vi "Test Create Report.vi"(8 "error in (no error)":errorcluster, 11 "XML Report Test in":refnum<class "Text Report Test.lvclass">) -> (0 "error out":errorcluster, 3 "XML Report Test out":refnum<class "Text Report Test.lvclass">)   [LabVIEW 2020, in "Text Report Test.lvclass"]
uses:
  Text Report Test.lvclass
  C:/Program Files (x86)/National Instruments/LabVIEW 2020/vi.lib/Astemes/LUnit/Test Case.lvclass
  Text Report Test.lvclass/Text Report Test.ctl
  <vilib>/Astemes/LUnit/Test Case.lvclass/Test Case.ctl
  <vilib>/Astemes/LUnit/Core/LUnit Test Case/Private/Append Fail Result.vi
  <vilib>/Astemes/LUnit/Core/LUnit Test Case/Private/Append Pass Result.vi
  <vilib>/Astemes/LUnit/Core/LUnit Test Case/Private/Run In UI.vi
  <vilib>/Utility/error.llb/Clear Errors.vi
  source/Plugins/Text Report/Text Report.lvclass
  <vilib>/Astemes/LUnit/Test Case.lvclass
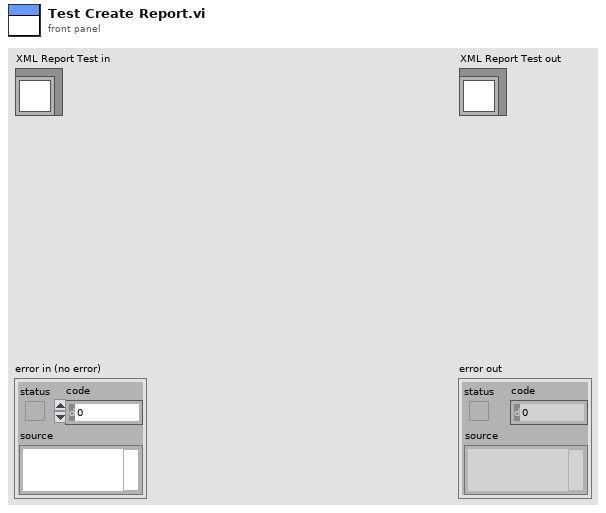
[diagram p1: front panel]
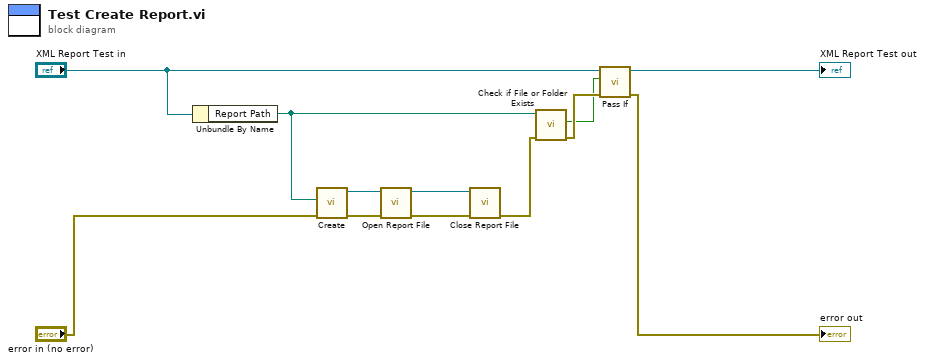
[diagram p0: block diagram]
diagram:
  n1 = Unbundle By Name("XML Report Test in") -> ("Report Path"=w1:path)
  n2 = call "Create.vi"("error in (no error)"="error in (no error)", "Report Path"=w1) -> ("error out"=w3:errorcluster, "Text Report"=w2:refnum<class "Text Report.lvclass">)  [unwired: 8 in]
  n3 = call-dynamic "Open Report File.vi"("error in (no error)"=w3, "Text Report In"=w2) -> ("error out"=w12:errorcluster, "Text Report Out"=w11:refnum<class "Text Report.lvclass">)  [unwired: 8 in]
  n4 = call-dynamic "Close Report File.vi"("error in (no error)"=w12, "Text Report In"=w11) -> ("error out"=w7:errorcluster)  [unwired: 8 in, 1 out]
  n5 = call <vilib>:"Check if File or Folder Exists.vi"("error in (no error)"=w7, "path"=w1) -> ("error out"=w6:errorcluster, "file or folder exists?"=w5:bool)  [unwired: 7 in, 1 out]
  n6 = call <vilib>:"Pass If.vi"("error in (no error)"=w6, "Pass?"=w5, "LUnit Test Case In"="XML Report Test in") -> ("error out"=→"error out":errorcluster, "LUnit Test Case Out"=→"XML Report Test out":refnum<class "Text Report Test.lvclass">)  [unwired: 7 in]
